vi "Example USB scanner.vi"(8 "error in (no error)":errorcluster) -> (0 "error out":errorcluster, 2 "Execution time":u32, 3 "USB devices":T1(array[cluster]))   [LabVIEW 2018]
uses:
  System.Management
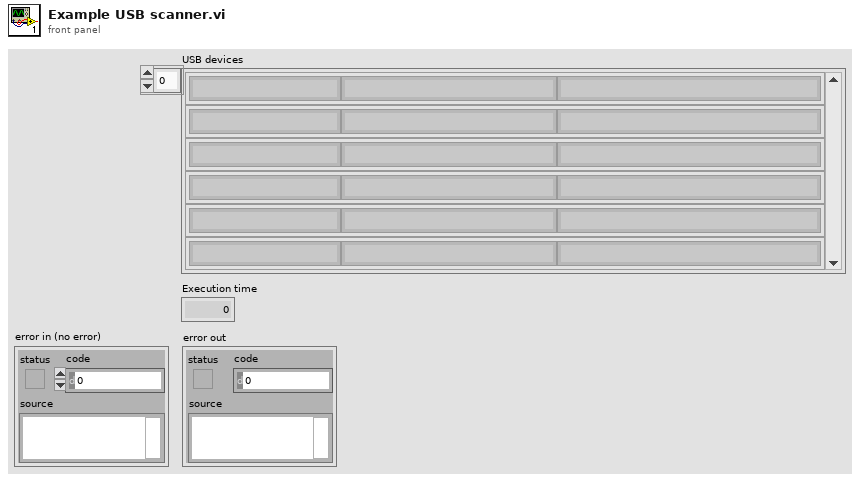
[diagram p1: front panel]
types:
  T1 = cluster{"[0]":string, "[1]":string, "[2]":string}[]
  T2 = cluster{"[0]":string, "[1]":string, "[2]":string}
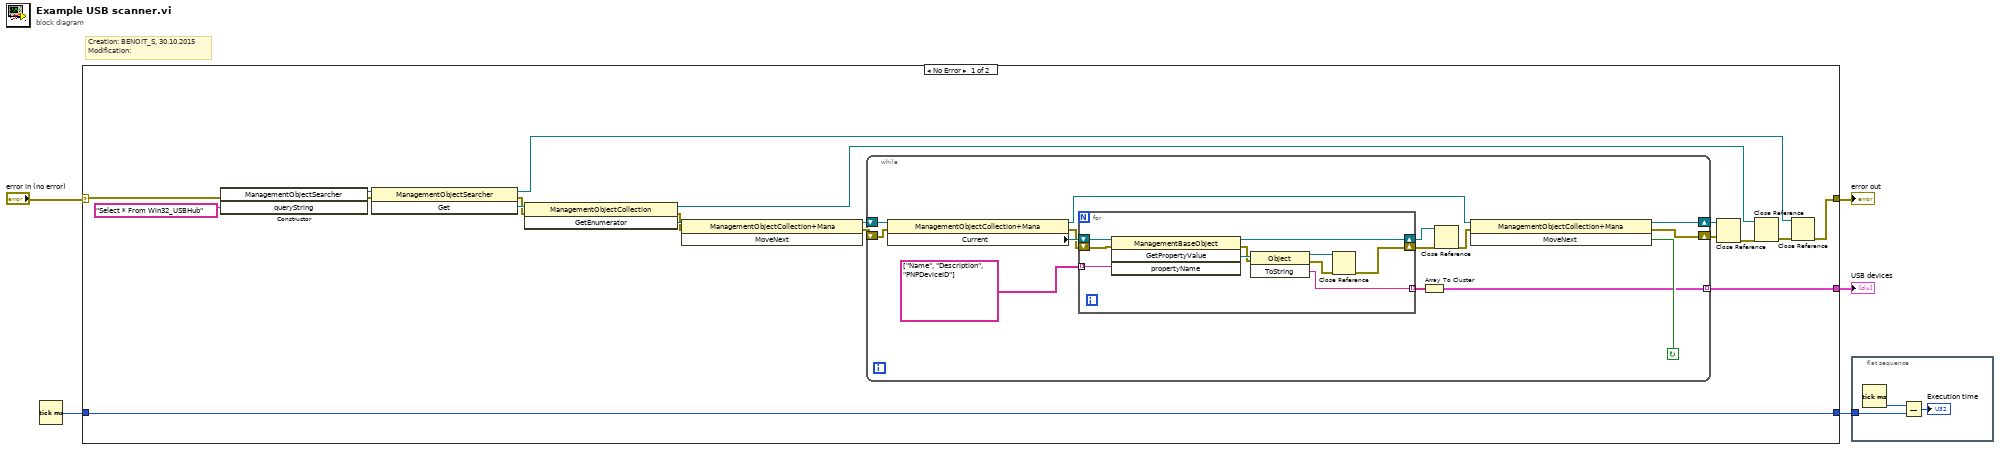
[diagram p0: block diagram]
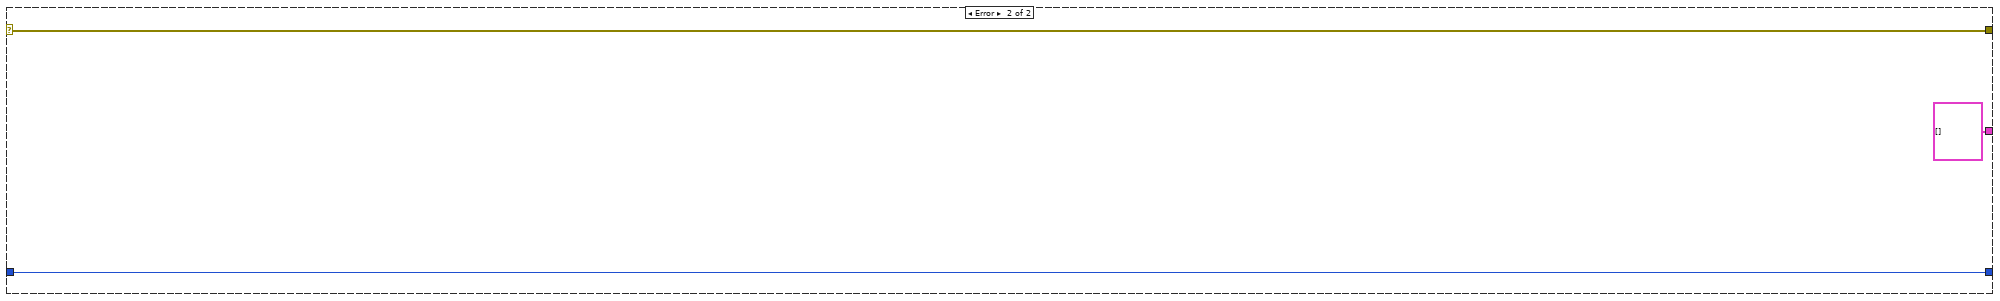
[diagram p2: hidden frame]
diagram:
  # "Creation: BENOIT_S, 30.10.2015\nModification:"
  n1 = Tick Count (ms)() -> (millisecond timer value=w2:u32)
  n2 = case shown="No Error" "error in (no error)" {
    selector: "error in (no error)" -> [w7 w51]
    tunnel: [w9 w51] -> w5
    tunnel: [w8 T1 []] -> w4
    tunnel: w2 -> [w6 w50]
    tunnel: [w6 w50] -> w1
    frame No Error {
      n3 = constructor class="ManagementObjectSearcher"(error in=w7, "queryString"="Select * From Win32_USBHub") -> (reference out=w23:refnum<k24>, error out=w22:errorcluster)  [unwired: 2 in, 2 out]
      n4 = invoke class="ManagementObjectSearcher" method="Get"(reference=w23, error in=w22) -> (reference out=w10:refnum<k24>, error out=w20:errorcluster, "Get"=w21:refnum<k24>)  [unwired: 1 in]
      n5 = invoke class="ManagementObjectCollection" method="GetEnumerator"(reference=w21, error in=w20) -> (reference out=w12:refnum<k24>, error out=w18:errorcluster, "GetEnumerator"=w19:refnum<k24>)  [unwired: 1 in]
      n6 = invoke class="ManagementObjectCollection+Mana" method="MoveNext"(reference=w19, error in=w18) -> (reference out=w17:refnum<k24>, error out=w16:errorcluster)  [unwired: 1 in, 1 out]
      n7 = while {
        shift-right: [w26] -> w14
        shift-left: w17 -> [w38]
        shift-right: [w25] -> w15
        shift-left: w16 -> [w37]
        tunnel: [w27] -> w8 mode=indexing
        stop <- w29 continue-if-true
        n8 = property class="ManagementObjectCollection+Mana"(reference=w38, error in=w37) -> (reference out=w31:refnum<k24>, error out=w33:errorcluster, "Current"=w36:refnum<k24>)
        n9 = for {
          shift-right: [w40] -> w32
          shift-left: w33 -> [w48]
          shift-right: [w41] -> w34
          shift-left: w36 -> [w47]
          tunnel: string[] ["Name", "Description", "PNPDeviceID"] -> [w46] mode=indexing
          tunnel: [w39] -> w28 mode=indexing
          n10 = invoke class="ManagementBaseObject" method="GetPropertyValue"(reference=w47, error in=w48, "propertyName"=w46) -> (reference out=w41:refnum<k24>, error out=w42:errorcluster, "GetPropertyValue"=w45:refnum<k24>)  [unwired: 1 in, 1 out]
          n11 = invoke class="Object" method="ToString"(reference=w45, error in=w42) -> (reference out=w44:refnum<k24>, error out=w43:errorcluster, "ToString"=w39:string)  [unwired: 1 in]
          n12 = Close Reference(reference=w44, error in (no error)=w43) -> (error out=w40:errorcluster)
        }
        n13 = Array To Cluster(array=w28) -> (cluster=w27:T2)
        n14 = Close Reference(reference=w34, error in (no error)=w32) -> (error out=w30:errorcluster)
        n15 = invoke class="ManagementObjectCollection+Mana" method="MoveNext"(reference=w31, error in=w30) -> (reference out=w26:refnum<k24>, error out=w25:errorcluster, "MoveNext"=w29:bool)  [unwired: 1 in]
      }
      n16 = Close Reference(reference=w14, error in (no error)=w15) -> (error out=w13:errorcluster)
      n17 = Close Reference(reference=w12, error in (no error)=w13) -> (error out=w11:errorcluster)
      n18 = Close Reference(reference=w10, error in (no error)=w11) -> (error out=w9:errorcluster)
    }
    frame Error {
    }
  }
  "error out" <- w5
  "USB devices" <- w4
  n19 = flat-sequence {
    tunnel: w1 -> [w53]
    frame #0 {
      n20 = Tick Count (ms)() -> (millisecond timer value=w54:u32)
      n21 = Subtract(x=w54, y=w53) -> (x-y=→"Execution time":u32)
    }
  }
